vi "Create User Event Refnums.vi"(8 "error in (no error)":errorcluster) -> (0 "error out":errorcluster, 3 "User Events to TCP Engine":T1)   [LabVIEW 2016, in "SLL Easy API via TCP.lvclass"]
uses:
  SLL Easy API via TCP.lvclass
  _Typedefs/User Events to TCP Engine.ctl
  _Typedefs/TCP Event Data.ctl
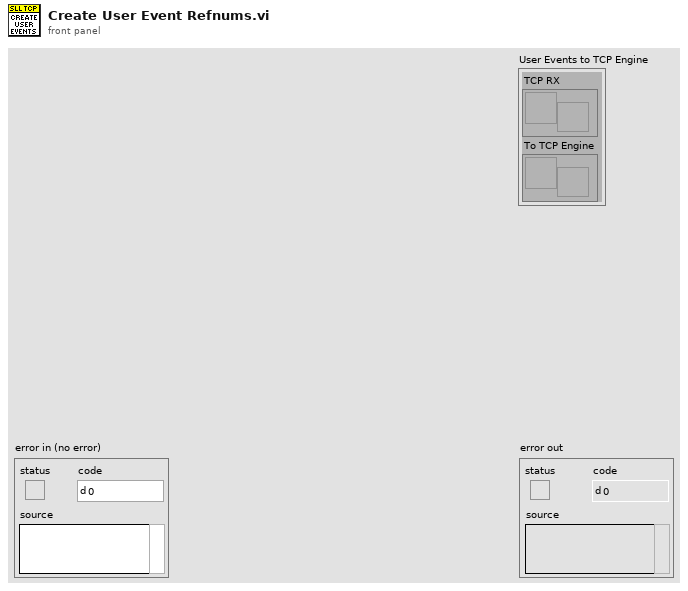
[diagram p1: front panel]
types:
  T1 = typedef "SLL Easy API via TCP.lvclass/User Events to TCP Engine.ctl" = cluster{"TCP RX":refnum<user-event>, "To TCP Engine":refnum<user-event>}
  T2 = typedef "SLL Easy API via TCP.lvclass/TCP Event Data.ctl" = cluster{"Connection ID":refnum<k5>, "String":string}
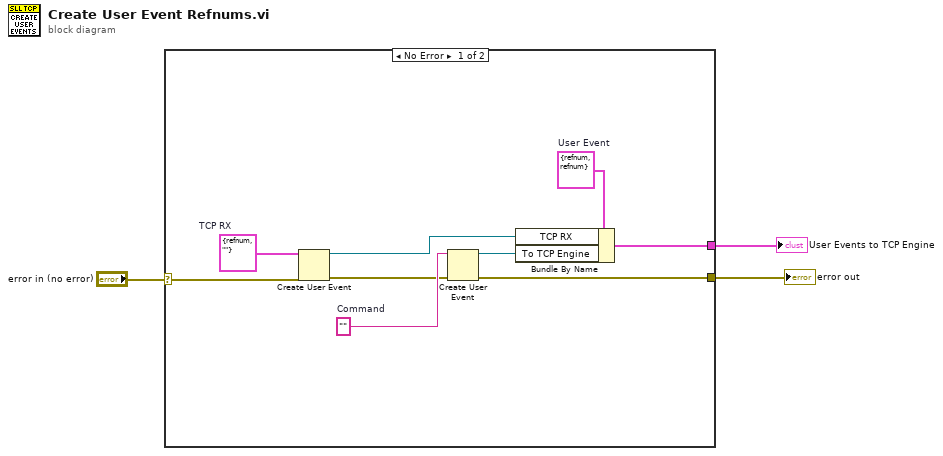
[diagram p0: block diagram]
diagram:
  n1 = case shown="No Error" "error in (no error)" {
    selector: "error in (no error)" -> [w4 w13]
    tunnel: [w8 _] -> w3
    tunnel: [w5 w13] -> w2
    frame No Error {
      w10 = T1 {"TCP RX"=refnum, "To TCP Engine"=refnum}  # User Event
      w12 = ""  # Command
      w7 = T2 {"Connection ID"=refnum, "String"=""}  # TCP RX
      n2 = Create User Event(user event datatype=w7, error in=w4) -> (user event=w6:refnum<user-event>, error out=w11:errorcluster)
      n3 = Create User Event(user event datatype=w12, error in=w11) -> (user event=w9:refnum<user-event>, error out=w5:errorcluster)
      n4 = Bundle By Name(cluster=w10, "TCP RX"=w6, "To TCP Engine"=w9) -> (w8:T1)
    }
    frame Error {
    }
  }
  "User Events to TCP Engine" <- w3
  "error out" <- w2
